vi "Enqueue Message.vi"(6 "Priority":bool, 8 "Error In":errorcluster, 9 "Data":variant, 10 "Command":string, 11 "Message Queue In":refnum<queue>) -> (0 "Error Out":errorcluster, 3 "Message Queue Out":refnum<queue>)   [LabVIEW 2017, in "Bookmark Manager.lvlib"]
uses:
  Bookmark Manager.lvlib
  Message.ctl
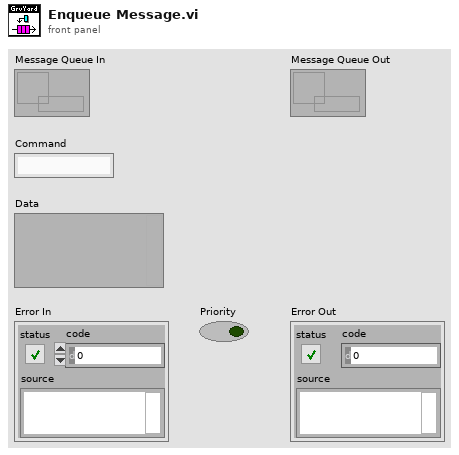
[diagram p1: front panel]
types:
  T1 = typedef "Bookmark Manager.lvlib/Message.ctl" = cluster{"Command":string, "Data":variant}
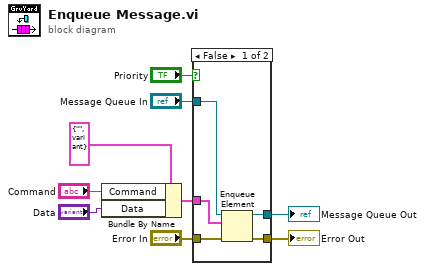
[diagram p0: block diagram]
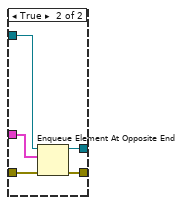
[diagram p2: hidden frame]
diagram:
  n1 = Bundle By Name(cluster=T1 {"Command"="", "Data"=variant} ("element"), "Command"="Command", "Data"="Data") -> (w5:T1)
  n2 = case shown="False" "Priority" {
    tunnel: "Message Queue In" -> [w14 w19]
    tunnel: w5 -> [w13 w17]
    tunnel: [w12 w18] -> w2
    tunnel: "Error In" -> [w11 w16]
    tunnel: [w10 w15] -> w3
    frame False {
      n3 = Enqueue Element(queue=w14, element=w13, error in (no error)=w11) -> (queue out=w12:refnum<queue>, error out=w10:errorcluster)  [unwired: 1 in, 1 out]
    }
    frame True {
      n4 = Enqueue Element At Opposite End(queue=w19, element=w17, error in (no error)=w16) -> (queue out=w18:refnum<queue>, error out=w15:errorcluster)  [unwired: 1 in, 1 out]
    }
  }
  "Error Out" <- w3
  "Message Queue Out" <- w2
